vi "Read Timeout Message Info.vi"(11 "IEventHandler in":refnum<class "IEventHandler.lvclass">) -> (0 "Timeout Message Priority":T1=enum."Normal", 1 "Timeout Message":refnum<class "Message.lvclass">, 2 "EventAggregator Enqueuer":refnum<class "Message Enqueuer.lvclass">, 3 "Timeout [ms]":i32)   [LabVIEW 2017, in "ActorEvents.lvlib" / "IEventHandler.lvclass"]
uses:
  IEventHandler.lvclass
  <vilib>/ActorFramework/Message Enqueuer/Message Enqueuer.lvclass
  <vilib>/ActorFramework/Message/Message.lvclass
  <vilib>/ActorFramework/Message Enqueuer/Message Priority.ctl
  IEventHandler.lvclass/IEventHandler.ctl
panel:
  # "Use property nodes"
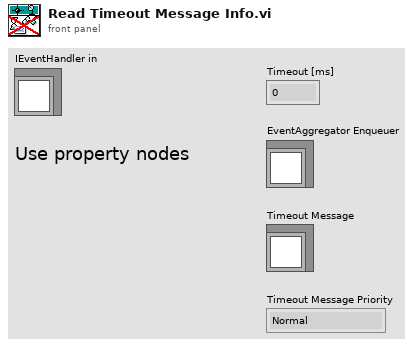
[diagram p1: front panel]
types:
  T1 = typedef "Actor Framework.lvlib/Message Enqueuer.lvclass/Message Priority.ctl" = enum16{"Low", "Normal", "High"}
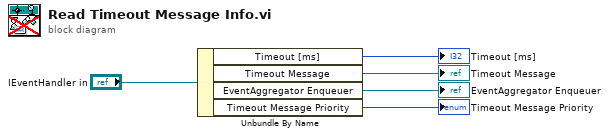
[diagram p0: block diagram]
diagram:
  n1 = Unbundle By Name("IEventHandler in") -> ("Timeout [ms]"=→"Timeout [ms]":i32, "Timeout Message"=→"Timeout Message":refnum<class "Message.lvclass">, "EventAggregator Enqueuer"=→"EventAggregator Enqueuer":refnum<class "Message Enqueuer.lvclass">, "Timeout Message Priority"=→"Timeout Message Priority":T1)
